vi "CalForUpd_sub.vi"(5 "Con.F":i32=20, 6 "Relu(MeaVal)":dbl[](array[numeric]), 7 "Pattern_Y":i16=9, 8 "MNIST(x)":i32[][](array[numeric])) -> (0 "out(delta)":ext[](array[numeric]), 1 "Out(delta*X)":ext[][](array[numeric]), 2 "Output(SoftMax)":ext[](array[numeric]), 3 "Output(Converted)":dbl[](array[numeric]), 4 "Entropy":ext)   [LabVIEW 2021]
panel:
  out "Output (Converted)":dbl[](graph)=[39.62523093192144, 0.0, 23.097154266476934, 78.25935170802192, 80.61297751490206, 88.079328272374, 139.1328670628771, 91.58552612543261, 147.85235008560898, 50.15605743167636]
  out "Output (SoftMax)":ext[](graph)=[9.942335489197921718e-48, 6.1442556256622408318e-65, 6.5983587063865749592e-55, 5.9713685974966820238e-31, 6.2840637228245183395e-30, 1.0985896780412405855e-26, 0.000163344942582687903655, 3.6606473610987689061e-25, 0.99983665505741731205, 3.7236448483001870884e-43]
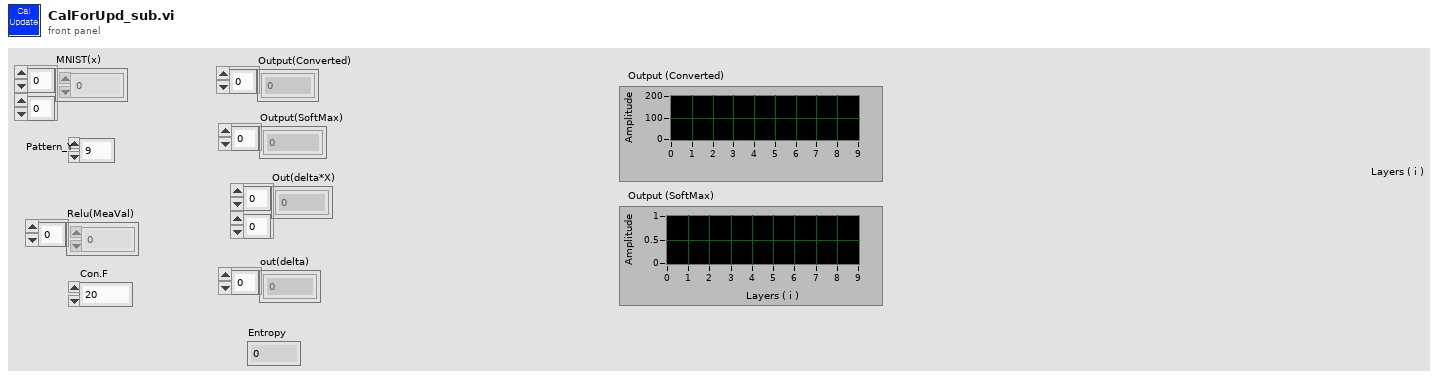
[diagram p1: front panel]
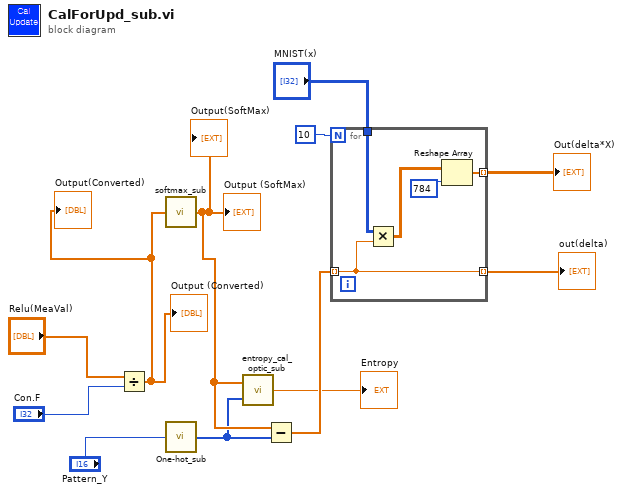
[diagram p0: block diagram]
diagram:
  n1 = Divide(x="Relu(MeaVal)", y="Con.F") -> (x/y=w8:dbl[])
  "Output (Converted)" <- w8
  "Output(Converted)" <- w8
  n2 = call "softmax_sub.vi"("Input"=w8) -> ("Output"=w7:ext[])
  "Output (SoftMax)" <- w7
  "Output(SoftMax)" <- w7
  n3 = call "One-hot_sub.vi"("Input(Y)"="Pattern_Y") -> ("Output(One-hot)"=w6:i32[])
  n4 = call "entropy_cal_optic_sub.vi"("T_1D"=w6, "Y_1D"=w7) -> ("Entropy"=→"Entropy":ext)
  n5 = Subtract(x=w7, y=w6) -> (x-y=w11:ext[])
  n6 = for {
    N: 10 -> [_]
    tunnel: w11 -> [w16] mode=indexing
    tunnel: [w16] -> w2 mode=indexing
    tunnel: [w15] -> w3 mode=indexing
    tunnel: "MNIST(x)" -> [w14]
    n7 = Multiply(x=w14, y=w16) -> (x*y=w13:ext[][])
    n8 = Reshape Array(w13, 784 ("차원 크기")) -> (w15:ext[])
  }
  "Out(delta*X)" <- w3
  "out(delta)" <- w2
